vi "Detect Finger.vi"(0 "VISA Refnum in":refnum<visa-resource-name>, 2 "Cmd":string="ï\u0001ÿÿÿÿ\u0001\u0000\u0003\u0001\u0000\u0005", 11 "error in (no error)":errorcluster, 12 "Buffer In":string) -> (3 "ID":i16, 4 "VISA Refnum out":refnum<visa-resource-name>, 8 "Response":string, 13 "Cmd Suceed?":bool, 14 "Buffer Out":string, 15 "error out":errorcluster)   [LabVIEW 2020]
uses:
  <vilib>/Instr/_visa.llb/VISA Flush IO Buffer Mask.ctl
panel:
  out "Confirmation Code":string
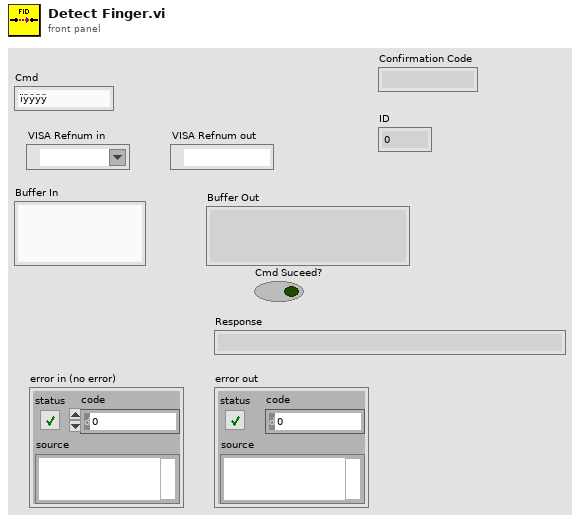
[diagram p1: front panel]
types:
  T1 = typedef "VISA Flush IO Buffer Mask.ctl" = u16
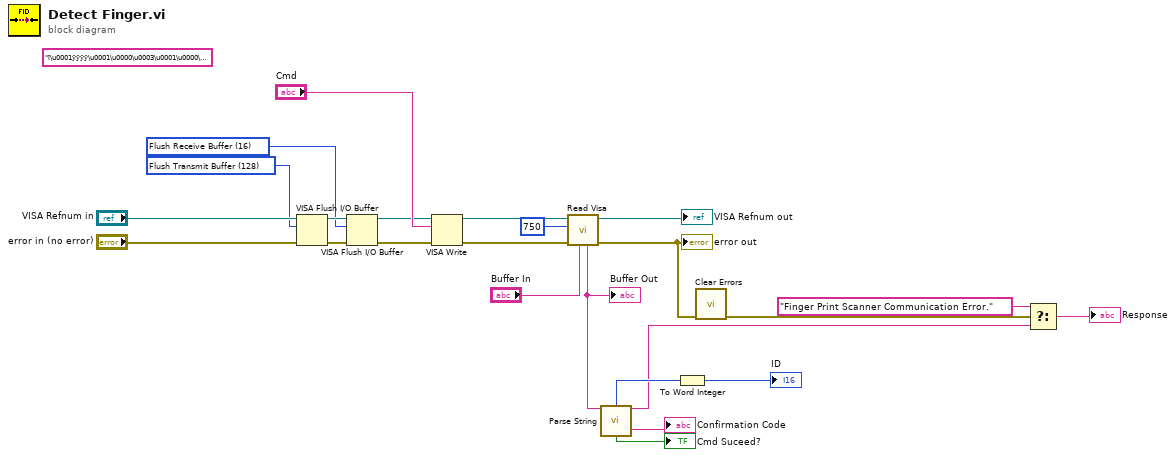
[diagram p0: block diagram]
diagram:
  (unwired) "ï\u0001ÿÿÿÿ\u0001\u0000\u0003\u0001\u0000\u0005" ("write buffer")
  w11 = T1 16 items=["Flush Receive Buffer"=16, "Write Transmit Buffer to Device"=32, "Flush Receive Buffer (No I/O)"=64, "Flush Transmit Buffer"=128] ("Mask")
  w16 = T1 128 items=["Flush Receive Buffer"=16, "Write Transmit Buffer to Device"=32, "Flush Receive Buffer (No I/O)"=64, "Flush Transmit Buffer"=128] ("Mask")
  n1 = VISA Flush I/O Buffer(VISA resource name="VISA Refnum in", mask (16)=w16, error in (no error)="error in (no error)") -> (VISA resource name out=w13:refnum<visa-resource-name>, error out=w15:errorcluster)
  n2 = VISA Flush I/O Buffer(VISA resource name=w13, mask (16)=w11, error in (no error)=w15) -> (VISA resource name out=w12:refnum<visa-resource-name>, error out=w14:errorcluster)
  n3 = VISA Write(VISA resource name=w12, write buffer="Cmd", error in (no error)=w14) -> (VISA resource name out=w19:refnum<visa-resource-name>, error out=w20:errorcluster)  [unwired: 1 out]
  n4 = call <userlib>:"Read Visa.vi"("Buffer In"="Buffer In", "error in (no error)"=w20, "delay before read (ms)"=u32 750, "VISA Refnum in"=w19) -> ("error out"=w5:errorcluster, "VISA Refnum out"=→"VISA Refnum out":refnum<visa-resource-name>, "Buffer Out"=w24:string)  [unwired: 5 in]
  "Buffer Out" <- w24
  "error out" <- w5
  n5 = call "Parse String.vi"("Ack package"=w24) -> ("Page ID"=w8:u16, "Ackmnt"=w4:string, "Cmd Suceed?"=→"Cmd Suceed?":bool, "Confirmation Code"=→"Confirmation Code":string)  [unwired: 11 in]
  n6 = To Word Integer(number=w8) -> (16bit integer=→"ID":i16)
  n7 = call <vilib>:"Clear Errors.vi"("error in (no error)"=w5) -> ("error out"=w1:errorcluster)  [unwired: 5 in, 1 out]
  n8 = Select(t="Finger Print Scanner Communication Error.", s=w1, f=w4) -> (s? t:f=→"Response":string)
